vi "ReadallDevicesv2.vi"(0 "GPIB HP 2":string="13", 1 "HP 2":bool, 2 "AH":bool=TRUE, 3 "GPIB HP":string="14", 4 "HP 1":bool=TRUE, 5 "error in":T1, 6 "LI 3":bool, 7 "GPIB L 3":string="8", 9 "TempSensor":bool, 10 "LI 2":bool, 11 "GPIB L 2":string="8", 12 "LI 1":bool, 13 "GPIB L 1":string="8", 14 "Nr. of Accumulations":i32=5, 17 "Y-Axis Field (kG)":dbl, 18 "Radial (r) Field (kG) 2":dbl) -> (15 "appended array":dbl[](array[numeric]), 19 "error out":errorcluster)   [LabVIEW 2009]
panel:
  in  "GPIB SIM900":string="2"
  in  "Port Num- TRBridge":string="7"
  out "Messfile Refnum":refnum<file>
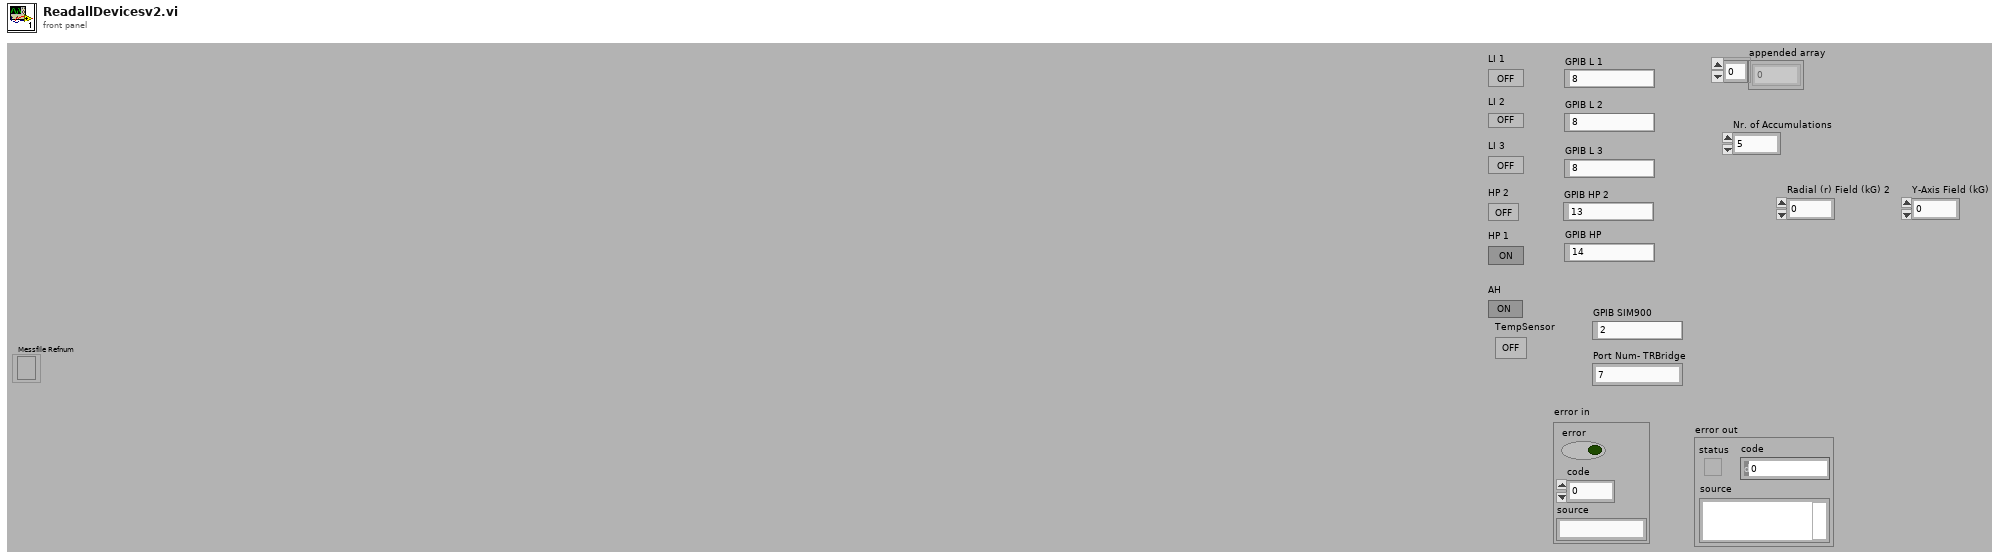
[diagram p1: front panel]
types:
  T1 = cluster{"error":bool, "code":i32, "source":string}
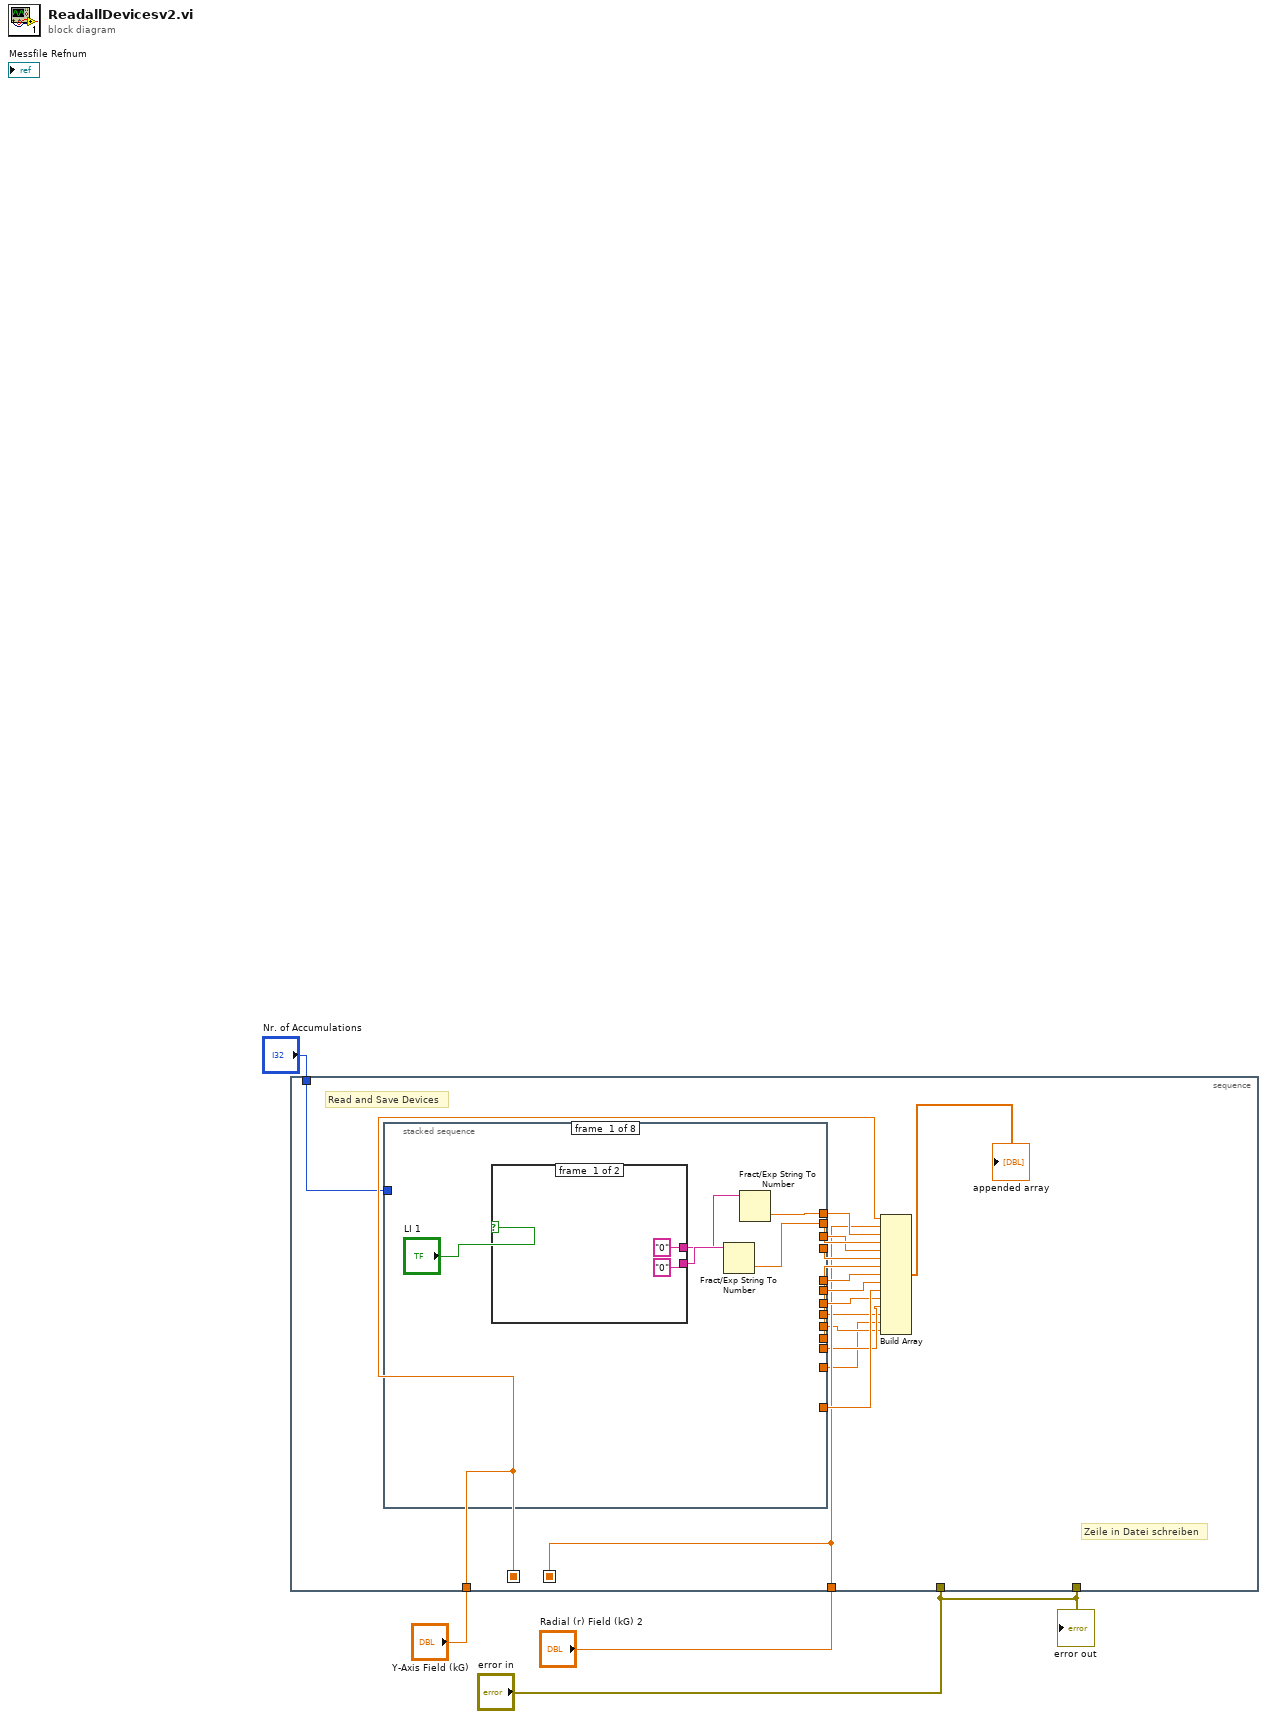
[diagram p0: block diagram]
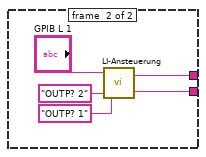
[diagram p2: hidden frame]
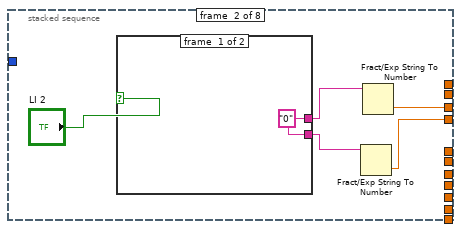
[diagram p3: hidden frame]
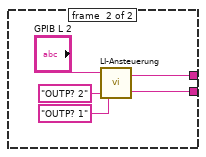
[diagram p4: hidden frame]
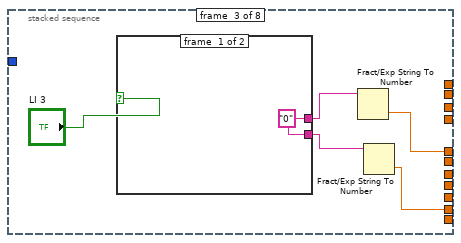
[diagram p5: hidden frame]
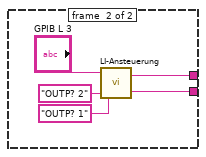
[diagram p6: hidden frame]
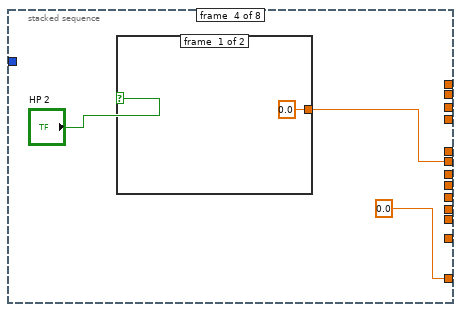
[diagram p7: hidden frame]
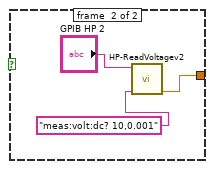
[diagram p8: hidden frame]
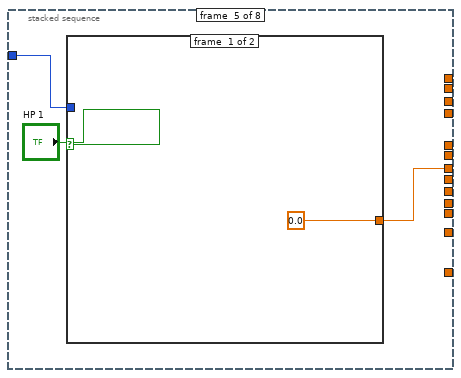
[diagram p9: hidden frame]
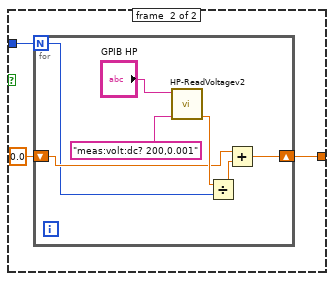
[diagram p10: hidden frame]
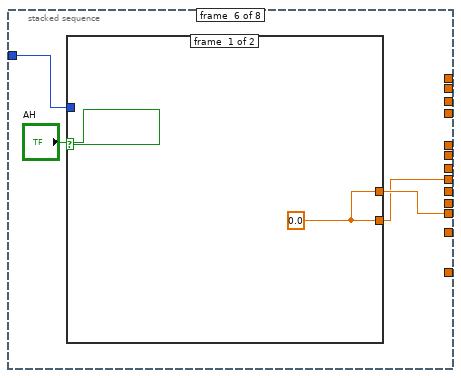
[diagram p11: hidden frame]
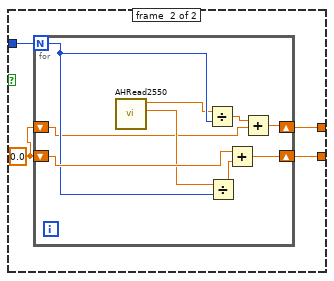
[diagram p12: hidden frame]
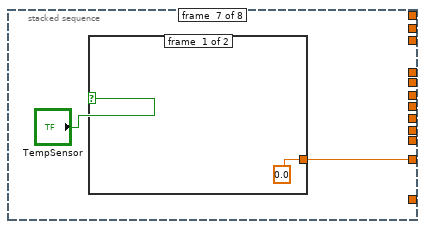
[diagram p13: hidden frame]
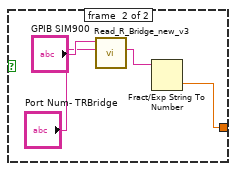
[diagram p14: hidden frame]
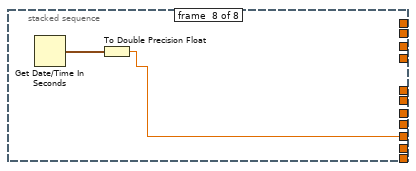
[diagram p15: hidden frame]
diagram:
  n1 = stacked-sequence {
    seq-local: [w10] -> [_]
    seq-local: [w11] -> [_]
    tunnel: "error in" -> [_]
    tunnel: "Y-Axis Field (kG)" -> [w11]
    tunnel: "Radial (r) Field (kG) 2" -> [w10]
    tunnel: "error in" -> [_]
    tunnel: "Nr. of Accumulations" -> [w9]
    frame #0 {
      # "Zeile in Datei schreiben"
      # "Read and Save Devices"
      n2 = stacked-sequence {
        tunnel: [w23 _ _ _ _ _ _ _] -> w21
        tunnel: [w22 _ _ _ _ _ _ _] -> w20
        tunnel: [_ w36 _ _ _ _ _ _] -> w19
        tunnel: [_ w34 _ _ _ _ _ _] -> w18
        tunnel: [_ _ w46 _ _ _ _ _] -> w17
        tunnel: [_ _ w45 _ _ _ _ _] -> w16
        tunnel: [_ _ _ w57 _ _ _ _] -> w15
        tunnel: [_ _ _ 0.0 _ _ _ _] -> w14
        tunnel: [_ _ _ _ w64 _ _ _] -> w13
        tunnel: [_ _ _ _ _ _ _ w102] -> w6
        tunnel: w9 -> [_ _ _ _ w63 w79 _ _]
        tunnel: [_ _ _ _ _ w78 _ _] -> w8
        tunnel: [_ _ _ _ _ w77 _ _] -> w7
        tunnel: [_ _ _ _ _ _ w95 _] -> w5
        frame #0 {
          n3 = case shown="True" "LI 1" {
            tunnel: ["0" ("Antwort2") w30] -> w25
            tunnel: ["0" ("Antwort1") w29] -> w24
            frame #0 {
            }
            frame #1 {
              n4 = call "LI-Ansteuerung.vi"("Frage2"="OUTP? 2", "Frage1"="OUTP? 1", "address string"="GPIB L 1") -> ("Antwort2"=w30:string, "Antwort1"=w29:string)
            }
          }
          n5 = Fract/Exp String To Number(string=w25) -> (number=w22:dbl)  [unwired: 3 in, 1 out]
          n6 = Fract/Exp String To Number(string=w24) -> (number=w23:dbl)  [unwired: 3 in, 1 out]
        }
        frame #1 {
          n7 = case shown="True" "LI 2" {
            tunnel: [w39 w41] -> w35
            tunnel: [w39 w40] -> w37
            frame #0 {
              w39 = "0" ("Antwort1")
            }
            frame #1 {
              n8 = call "LI-Ansteuerung.vi"("Frage2"="OUTP? 2", "Frage1"="OUTP? 1", "address string"="GPIB L 2") -> ("Antwort2"=w41:string, "Antwort1"=w40:string)
            }
          }
          n9 = Fract/Exp String To Number(string=w35) -> (number=w34:dbl)  [unwired: 3 in, 1 out]
          n10 = Fract/Exp String To Number(string=w37) -> (number=w36:dbl)  [unwired: 3 in, 1 out]
        }
        frame #2 {
          n11 = case shown="True" "LI 3" {
            tunnel: [w50 w52] -> w47
            tunnel: [w50 w51] -> w48
            frame #0 {
              w50 = "0" ("Antwort1")
            }
            frame #1 {
              n12 = call "LI-Ansteuerung.vi"("Frage2"="OUTP? 2", "Frage1"="OUTP? 1", "address string"="GPIB L 3") -> ("Antwort2"=w52:string, "Antwort1"=w51:string)
            }
          }
          n13 = Fract/Exp String To Number(string=w48) -> (number=w46:dbl)  [unwired: 3 in, 1 out]
          n14 = Fract/Exp String To Number(string=w47) -> (number=w45:dbl)  [unwired: 3 in, 1 out]
        }
        frame #3 {
          n15 = case shown="True" "HP 2" {
            tunnel: [0.0 ("Voltage") w60] -> w57
            frame #0 {
            }
            frame #1 {
              n16 = call "HP-ReadVoltagev2.vi"("String"="meas:volt:dc? 10,0.001", "HP-Mulitmeter\nGPIB Address"="GPIB HP 2") -> ("Voltage"=w60:dbl)  [unwired: 9 in]
            }
          }
        }
        frame #4 {
          n17 = case shown="True" "HP 1" {
            tunnel: [0.0 ("Voltage") w69] -> w64
            tunnel: w63 -> [_ w68]
            frame #0 {
            }
            frame #1 {
              n18 = for {
                N: w68 -> [w70]
                shift-right: [w72] -> w69
                shift-left: 0.0 -> [w71]
                n19 = call "HP-ReadVoltagev2.vi"("String"="meas:volt:dc? 200,0.001", "HP-Mulitmeter\nGPIB Address"="GPIB HP") -> ("Voltage"=w74:dbl)  [unwired: 9 in]
                n20 = Divide(x=w74, y=w70) -> (x/y=w73:dbl)
                n21 = Add(x=w71, y=w73) -> (x+y=w72:dbl)
              }
            }
          }
        }
        frame #5 {
          n22 = case shown="True" "AH" {
            tunnel: [w81 w85] -> w77
            tunnel: w79 -> [_ w84]
            tunnel: [w81 w82] -> w78
            frame #0 {
              w81 = 0.0 ("Voltage")
            }
            frame #1 {
              w83 = 0.0
              n23 = for {
                N: w84 -> [w90]
                shift-right: [w93] -> w85
                shift-left: w83 -> [w92]
                shift-right: [w86] -> w82
                shift-left: w83 -> [w87]
                n24 = call "AHRead2550.vi"() -> ("loss"=w91:dbl, "capacitance"=w89:dbl)  [unwired: 9 in, 1 out]
                n25 = Divide(x=w89, y=w90) -> (x/y=w88:dbl)
                n26 = Divide(x=w91, y=w90) -> (x/y=w94:dbl)
                n27 = Add(x=w92, y=w94) -> (x+y=w93:dbl)
                n28 = Add(x=w88, y=w87) -> (x+y=w86:dbl)
              }
            }
          }
        }
        frame #6 {
          n29 = case shown="True" "TempSensor" {
            tunnel: [0.0 ("Voltage") w98] -> w95
            frame #0 {
            }
            frame #1 {
              n30 = call "Read_R_Bridge_new_v3.vi"("Port Num- TRBridge"="Port Num- TRBridge", "GPIB-Adress"="GPIB SIM900") -> ("R out"=w99:string)  [unwired: 8 in, 1 out]
              n31 = Fract/Exp String To Number(string=w99) -> (number=w98:dbl)  [unwired: 3 in, 1 out]
            }
          }
        }
        frame #7 {
          n32 = Get Date/Time In Seconds() -> (seconds since 1Jan1904=w103:timestamp)
          n33 = To Double Precision Float(number=w103) -> (double precision float=w102:dbl)
        }
      }
      n34 = Build Array(w11, w10, w21, w20, w19, w18, w16, w17, w15, w14, w13, w8, w7, w5, w6) -> (→"appended array":dbl[])
    }
  }
  "error out" <- "error in"
